vi "setSpeed.vi"(6 "Delay between send and receive [ms]":i32=1000, 8 "error in (no error)":errorcluster, 10 "speed token":u16, 11 "CCD in":refnum<class "CCD.lvclass">) -> (0 "error out":errorcluster, 1 "ID":i32, 2 "results-JSON string":string, 3 "CCD out":refnum<class "CCD.lvclass">)   [LabVIEW 2023, in "CCD.lvclass"]
uses:
  CCD.lvclass
  20f7d3bd-08ac-4524-9bed-df36c1da25a0.vi
  cab240a6-cbf4-4e2c-ab79-96d9c1b88265.vi
  <vilib>/JDP Science/JSONtext/Variant to JSON Text.vi
  <vilib>/JDP Science/JSONtext/Set Item.vi
  <vilib>/JDP Science/JSONtext/LVClass Serializer/JSONtext LVClass Serializer.lvclass
  GenericDevice/GenericDevice.lvclass
  <vilib>/IlluminatedG/lv-web-crypto/lv-json/JSON/JSON.lvlib
panel:
  # "Connector Pane"
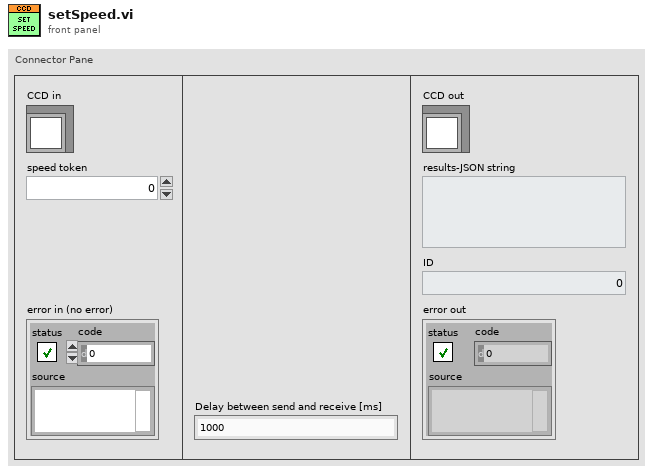
[diagram p1: front panel]
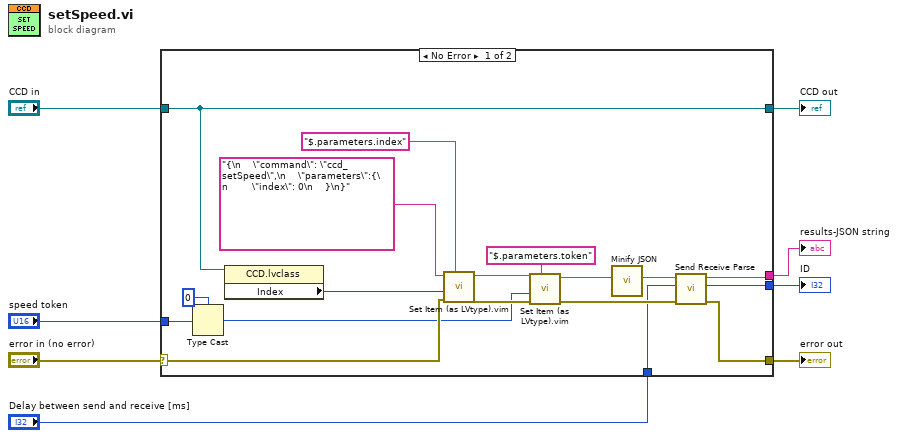
[diagram p0: block diagram]
diagram:
  n1 = case shown="No Error" "error in (no error)" {
    selector: "error in (no error)" -> [w22 w28]
    tunnel: [w17 w28] -> w7
    tunnel: [w24 w27] -> w5
    tunnel: "CCD in" -> [w24 w27]
    tunnel: [w16 _] -> w4
    tunnel: [w15 _] -> w3
    tunnel: "Delay between send and receive [ms]" -> [w12 _]
    tunnel: "speed token" -> [w11 _]
    frame No Error {
      n2 = Type Cast(type=u16 0, x=w11) -> (*(type *) &x=w9:u16)
      n3 = property class="CCD.lvclass"(reference=w24) -> ("Index"=w23:i32)  [unwired: 1 in, 2 out]
      n4 = call "Set Item (as LVtype).vim"("$Path or Item Name"="$.parameters.index", "error in (no error)"=w22, "Anything"=w23, "JSON"="{\n    \"command\": \"ccd_setSpeed\",\n    \"parameters\":{\n        \"index\": 0\n    }\n}") -> ("error out"=w20:errorcluster, "<JSON>"=w18:string)  [unwired: 4 in, 1 out]
      n5 = call "Set Item (as LVtype).vim"("$Path or Item Name"="$.parameters.token", "error in (no error)"=w20, "Anything"=w9, "JSON"=w18) -> ("error out"=w19:errorcluster, "<JSON>"=w14:string)  [unwired: 4 in, 1 out]
      n6 = call <vilib>:"Minify JSON.vi"("JSON String"=w14) -> ("Minified JSON"=w13:string)  [unwired: 10 in]
      n7 = call "Send Receive Parse.vi"("error in"=w19, "Delay between send and receive [ms]"=w12, "<JSON>"=w13) -> ("error out"=w17:errorcluster, "ID"=w15:i32, "results-JSON string"=w16:string)  [unwired: 6 in]
    }
    frame Error {
    }
  }
  "error out" <- w7
  "CCD out" <- w5
  "results-JSON string" <- w4
  "ID" <- w3
